vi "Find and Replace GObj.vi"(5 "GObj Class Name":string, 6 "GObj Label":string, 7 "Traverse Target":T1, 8 "error in (no error)":errorcluster, 9 "Case Insensitive Match? (F)":bool, 10 "Class Path":path, 11 "vi reference in":refnum<vi>) -> (0 "error out":errorcluster, 2 "Replace":refnum<vi>, 3 "vi reference out":refnum<vi>)   [LabVIEW 2020, in "Message Maker.lvlib"]
uses:
  Message Maker.lvlib
  <vilib>/Utility/traverseref.llb/TRef TravTarget.ctl
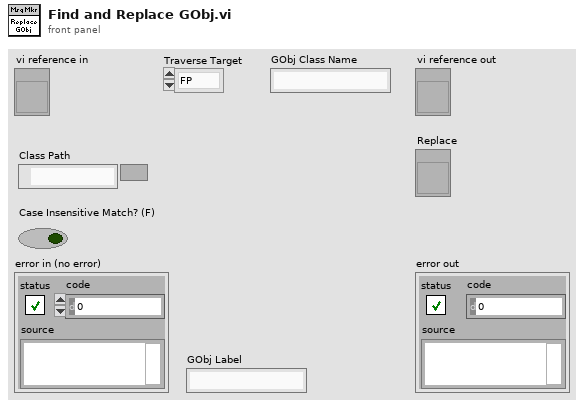
[diagram p1: front panel]
types:
  T1 = typedef "TRef TravTarget.ctl" = enum16{"FP", "BD", "Other"}
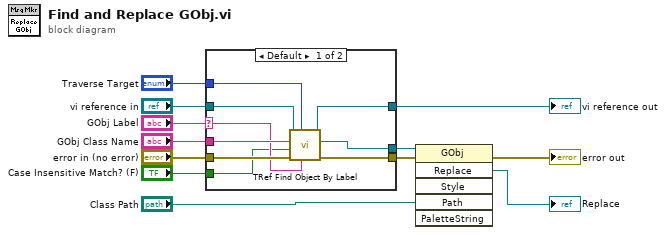
[diagram p0: block diagram]
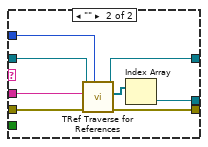
[diagram p2: hidden frame]
diagram:
  n1 = case shown="Default" "GObj Label" {
    selector: "GObj Label" -> [w15 _]
    tunnel: [w20 w29] -> w12
    tunnel: [w14 w28] -> w10
    tunnel: "GObj Class Name" -> [w16 w26]
    tunnel: "Traverse Target" -> [w19 w25]
    tunnel: [w17 w24] -> w7
    tunnel: "vi reference in" -> [w18 w23]
    tunnel: "error in (no error)" -> [w21 w22]
    tunnel: "Case Insensitive Match? (F)" -> [w13 _]
    frame Default {
      n2 = call <vilib>:"TRef Find Object By Label.vi"("Label"=w15, "Traverse Target"=w19, "error in (no error)"=w21, "Case Insensitive Match? (F)"=w13, "Class Name"=w16, "VI Ref"=w18) -> ("error out"=w20:errorcluster, "Found Obj Ref"=w14:refnum<vi>, "dup VI Ref"=w17:refnum<vi>)  [unwired: 2 in, 1 out]
    }
    frame "" {
      n3 = call <vilib>:"TRef Traverse for References.vi"("Traverse Target"=w25, "error in (no error)"=w22, "Class Name"=w26, "VI Refnum"=w23) -> ("error out"=w29:errorcluster, "References"=w27:refnum<vi>[], "dup VI Refnum"=w24:refnum<vi>)  [unwired: 4 in, 1 out]
      n4 = Index Array(array=w27) -> (element=w28:refnum<vi>)  [unwired: 1 in]
    }
  }
  "vi reference out" <- w7
  n5 = invoke class="GObj" method="Replace"(reference=w10, error in=w12, "Path"="Class Path") -> (error out=→"error out":errorcluster, "Replace"=→"Replace":refnum<vi>)  [unwired: 3 in, 4 out]
